vi "mWmotor_Auto_adjust.vi"(6 "Set_value":dbl=140.185, 7 "EIP":dbl, 8 "error in (no error)":errorcluster, 9 "Enable":bool, 10 "Degrees To move":dbl=1.0, 11 "MW motor":refnum<visa-resource-name>) -> (0 "error out":errorcluster, 3 "VISA resource name out":refnum<visa-resource-name>)   [LabVIEW 2019]
panel:
  in  "Range (GHz)":dbl=0.006
  out "In Range?":bool
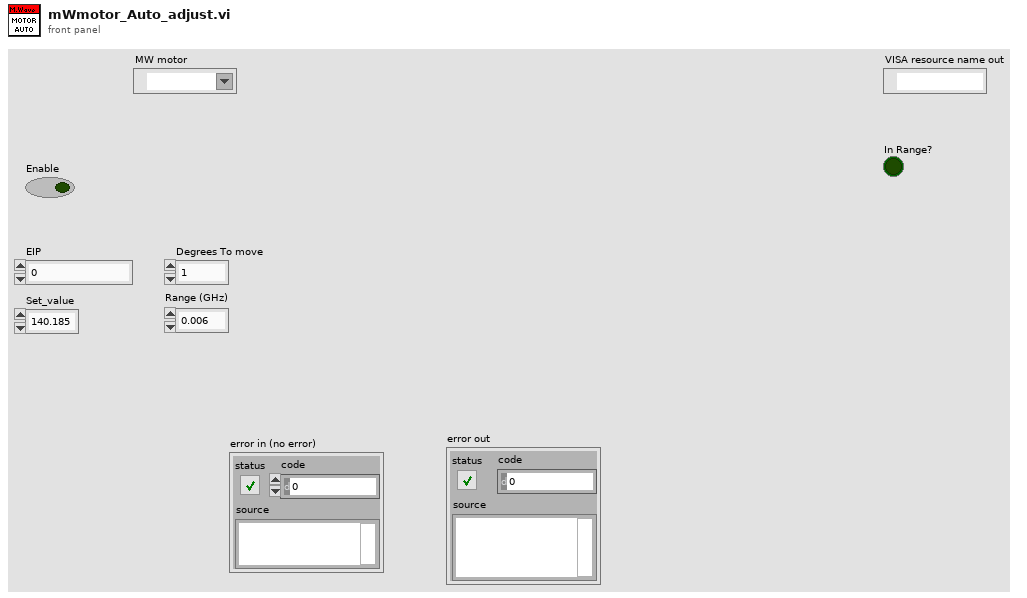
[diagram p1: front panel]
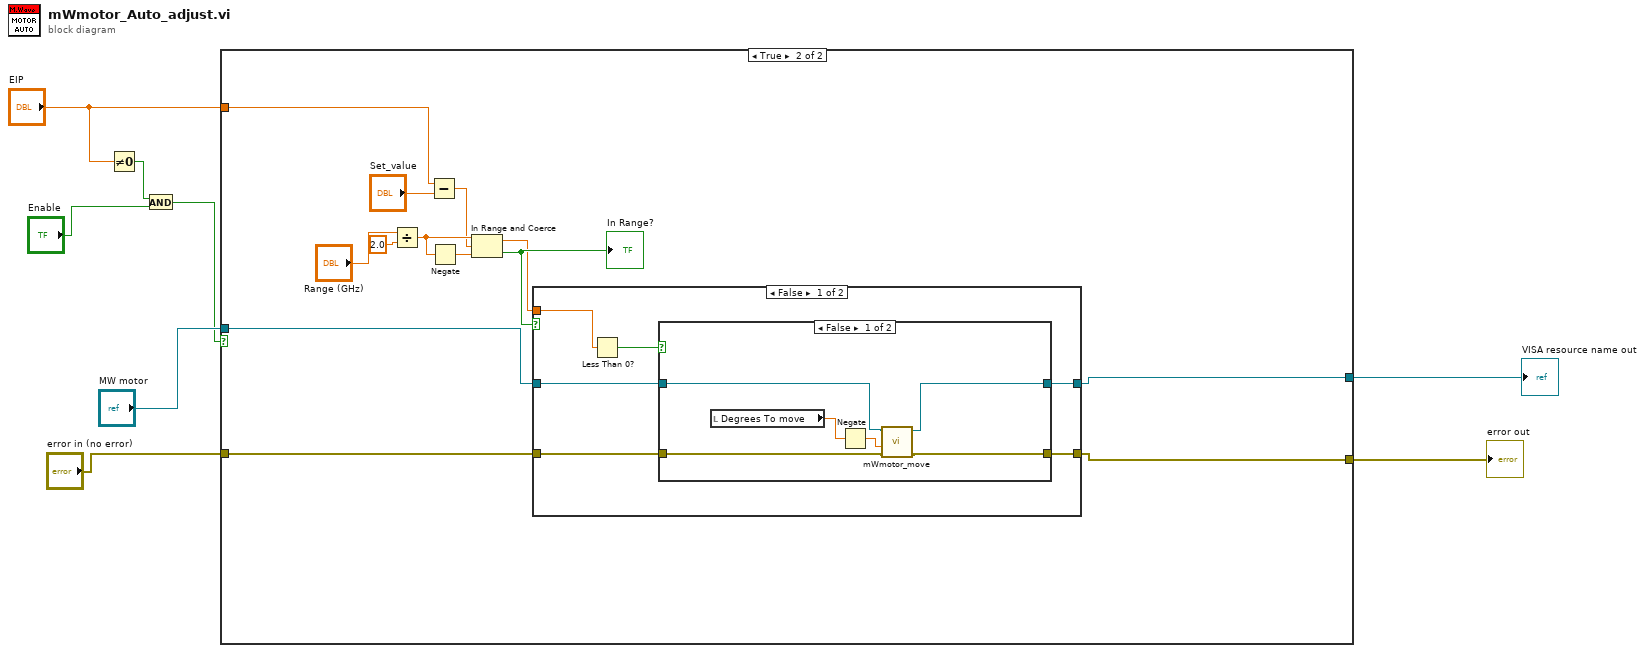
[diagram p0: block diagram]
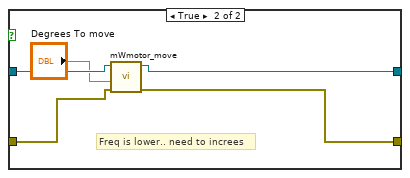
[diagram p3: hidden frame]
diagram:
  n1 = Not Equal To 0?(x="EIP") -> (x != 0?=w3:bool)
  n2 = And(x=w3, y="Enable") -> (x .and. y?=w1:bool)
  n3 = case shown="True" w1 {
    tunnel: [w9 w15] -> w8
    tunnel: [w10 w14] -> w7
    tunnel: "MW motor" -> [w10 w13]
    tunnel: "error in (no error)" -> [w9 w12]
    tunnel: "EIP" -> [_ w11]
    frame False {
    }
    frame True {
      n4 = Divide(x="Range (GHz)", y=2.0) -> (x/y=w21:dbl)
      n5 = Subtract(x=w11, y="Set_value") -> (x-y=w19:dbl)
      n6 = Negate(x=w21) -> (-x=w18:dbl)
      n7 = In Range and Coerce(upper limit=w21, x=w19, lower limit=w18) -> (coerced(x)=w16:dbl, In Range?=w17:bool)
      "In Range?" <- w17
      n8 = case shown="False" w17 {
        tunnel: w16 -> [w29 _]
        tunnel: w13 -> [w27 w42]
        tunnel: [w26 w42] -> w14
        tunnel: w12 -> [w25 w41]
        tunnel: [w24 w41] -> w15
        frame False {
          n9 = Less Than 0?(x=w29) -> (x < 0?=w28:bool)
          n10 = case shown="False" w28 {
            tunnel: w27 -> [w33 w40]
            tunnel: [w31 w39] -> w26
            tunnel: w25 -> [w34 w38]
            tunnel: [w30 w37] -> w24
            frame False {
              n11 = local read "Degrees To move"() -> (w35:dbl)
              n12 = Negate(x=w35) -> (-x=w32:dbl)
              n13 = call "mWmotor_move.vi"("error in (no error)"=w34, "Degrees To move"=w32, "MW motor"=w33) -> ("error out"=w30:errorcluster, "VISA resource name out"=w31:refnum<visa-resource-name>)  [unwired: 7 in]
            }
            frame True {
              # "Freq is lower.. need to increes"
              n14 = call "mWmotor_move.vi"("error in (no error)"=w38, "Degrees To move"="Degrees To move", "MW motor"=w40) -> ("error out"=w37:errorcluster, "VISA resource name out"=w39:refnum<visa-resource-name>)  [unwired: 7 in]
            }
          }
        }
        frame True {
          # "Frequecy is in range"
        }
      }
    }
  }
  "error out" <- w8
  "VISA resource name out" <- w7
